vi "Get Param Info.vi"(0 "paramID":i32, 1 "paramType":i32, 2 "paramAvailable":i32, 3 "paramReadOnly":i32, 4 "paramMin":dbl, 5 "paramMax":dbl, 6 "paramDefault":dbl, 7 "error in (no error)":errorcluster) -> (20 "function return":i32, 21 "paramType out":i32, 22 "paramAvailable out":i32, 23 "paramReadOnly out":i32, 24 "paramMin out":dbl, 25 "paramMax out":dbl, 26 "paramDefault out":dbl, 27 "error out":errorcluster)   [LabVIEW 2020, in "ThorECU.lvlib"]
doc: "long GetParamInfo(const long paramID, long &paramType, long &paramAvailable, long &paramReadOnly, double &paramMin, double &paramMax, double &paramDefault);"
uses:
  ThorECU.lvlib
  ThorECU.dll
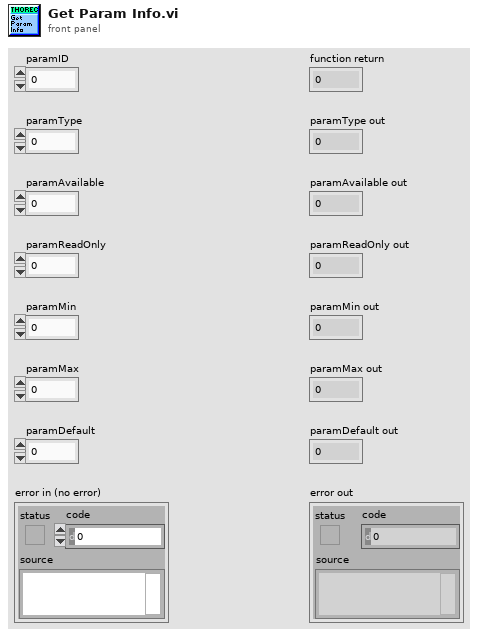
[diagram p1: front panel]
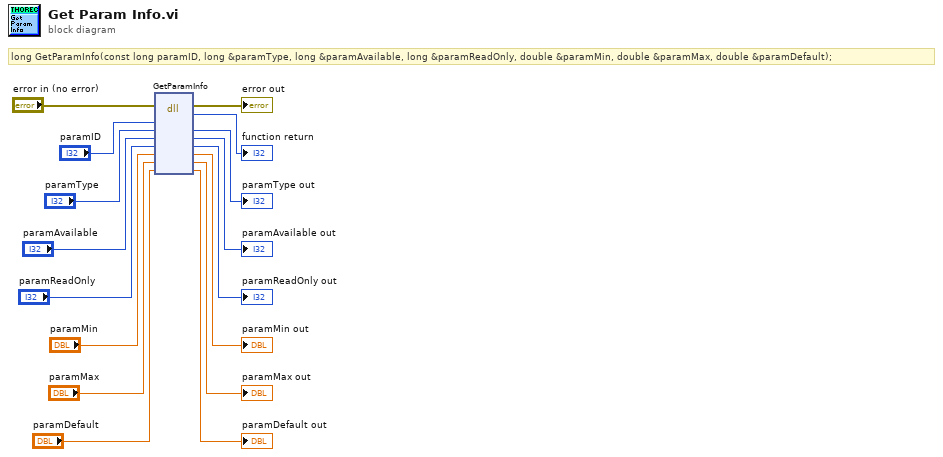
[diagram p0: block diagram]
diagram:
  # "long GetParamInfo(const long paramID, long &paramType, long &paramAvailable, long &paramReadOnly, double &paramMin, double &paramMax, double &paramDefault);"
  n1 = dll-call lib="D:/software/TweezerTron/ThorECU.*" fn="GetParamInfo"(error in="error in (no error)", "paramID"="paramID", "paramType"="paramType", "paramAvailable"="paramAvailable", "paramReadOnly"="paramReadOnly", "paramMin"="paramMin", "paramMax"="paramMax", "paramDefault"="paramDefault") -> (error out=→"error out":errorcluster, →"function return":i32, "paramType"=→"paramType out":i32, "paramAvailable"=→"paramAvailable out":i32, "paramReadOnly"=→"paramReadOnly out":i32, "paramMin"=→"paramMin out":dbl, "paramMax"=→"paramMax out":dbl, "paramDefault"=→"paramDefault out":dbl)  [unwired: 3 in, 1 out]
